vi "task 2.vi"() -> ()   [LabVIEW 2017]
panel:
  in  "max Voltage":dbl
  in  "Min Voltage":dbl
  in  "DAQmx Physical Channel":tag="Dev9/ao0"
  in  "Motor 1":dbl(slide) scale=0.0..10.0
  in  "stop":bool
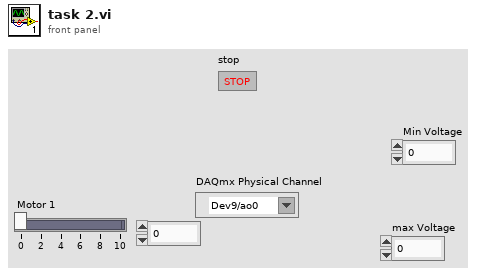
[diagram p1: front panel]
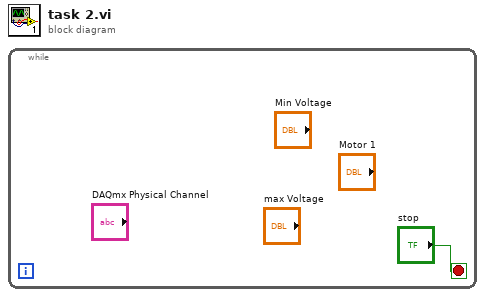
[diagram p0: block diagram]
diagram:
  n1 = while {
    stop <- "stop" stop-if-true
  }
